vi "Template_Test.vi"(8 "Numeric Control 4":dbl, 9 "Numeric Control 3":dbl, 10 "Numeric Control 2":dbl, 11 "Numeric Control":dbl) -> (0 "String":string, 1 "Numeric Indicator 3":dbl, 2 "Numeric Indicator 2":dbl, 3 "Numeric Indicator":dbl)   [LabVIEW 2014, in "Template.lvlib" / "Template_Class.lvclass"]
uses:
  Template_Class.lvclass
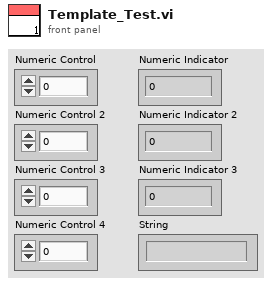
[diagram p1: front panel]
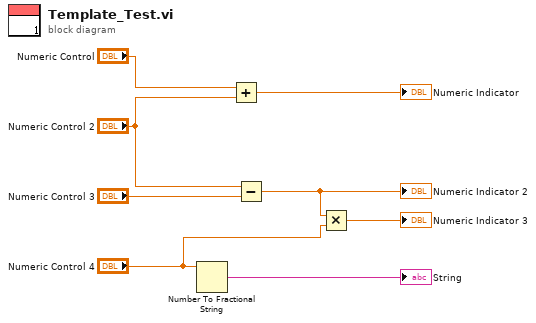
[diagram p0: block diagram]
diagram:
  n1 = Number To Fractional String(number="Numeric Control 4") -> (F-format string=→"String":string)  [unwired: 3 in]
  n2 = Add(x="Numeric Control", y="Numeric Control 2") -> (x+y=→"Numeric Indicator":dbl)
  n3 = Subtract(x="Numeric Control 2", y="Numeric Control 3") -> (x-y=w3:dbl)
  "Numeric Indicator 2" <- w3
  n4 = Multiply(x=w3, y="Numeric Control 4") -> (x*y=→"Numeric Indicator 3":dbl)
